vi "LED Lights Subsystem.vi"(8 "error in":errorcluster) -> ()   [LabVIEW 2015]
uses:
  <vilib>/Rock Robotics/SystemInterfaces/i2clib/i2c_bus.ctl
  <vilib>/Rock Robotics/Network Tables/NT Read Boolean.vi
panel:
  in  "Send":bool
  in  "Light ID":u8=3
  in  "Blue":u8=153
  in  "Green":u8=12
  in  "Red":u8=64
  out "error out":errorcluster
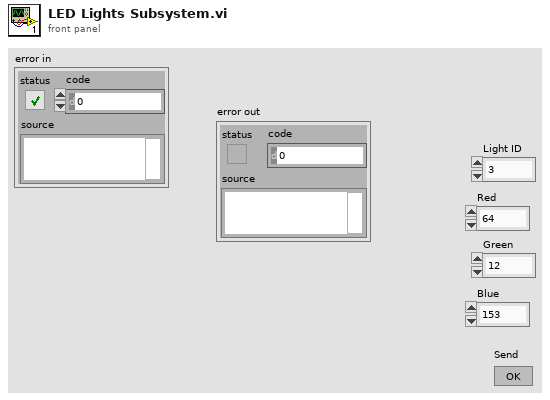
[diagram p1: front panel]
types:
  T1 = typedef "i2c_bus.ctl" = enum16{"I2C On-Board", "I2C MXP", "Invalid"}
  T2 = typedef "LED Lights Ref.ctl" = cluster{"I2CDevRef":T3}
  T3 = typedef "WPI_I2CDevRef.ctl" = cluster{"DevStatus":errorcluster, "Device Address":u8, "Handle":i32, "I2C Bus":T1}
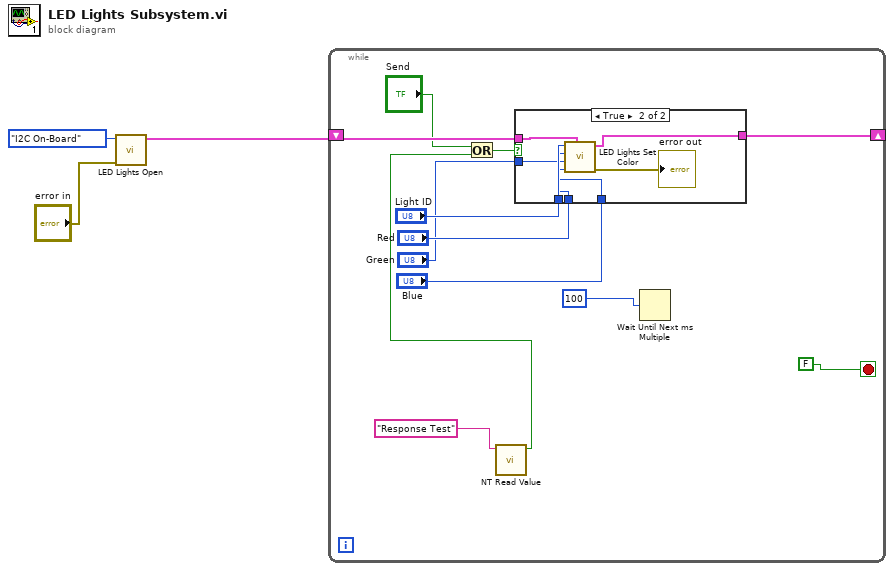
[diagram p0: block diagram]
diagram:
  n1 = call "LED Lights Open.vi"("error in"="error in", "I2C Bus"=i2c_bus."I2C On-Board") -> ("output cluster"=w2:T2)  [unwired: 8 in, 1 out]
  n2 = while {
    shift-right: [w8] -> _
    shift-left: w2 -> [w13]
    stop <- FALSE stop-if-true
    n3 = call-poly <vilib>:"NT Read Value.vi"("Name"="Response Test") -> ("Boolean"=w4:bool)  [unwired: 9 in, 1 out]
    n4 = Or(x="Send", y=w4) -> (x .or. y?=w7:bool)
    n5 = case shown="True" w7 {
      tunnel: w13 -> [w16 w23]
      tunnel: "Light ID" -> [_ w22]
      tunnel: "Red" -> [_ w21]
      tunnel: "Green" -> [_ w20]
      tunnel: "Blue" -> [_ w19]
      tunnel: [w16 w17] -> w8
      frame False {
      }
      frame True {
        n6 = call "LED Lights Set Color.vi"("LED Lights Ref In"=w23, "Blue"=w19, "Green"=w20, "Red"=w21, "Light ID"=w22) -> ("error out"=→"error out":errorcluster, "LED Lights Ref Out"=w17:T2)  [unwired: 5 in]
      }
    }
    n7 = Wait Until Next ms Multiple(millisecond multiple=100) -> ()  [unwired: 1 out]
  }
